vi "SMO.Example.DVRtoRef.vi"(10 "Ref":T1) -> (2 "Ref":u32 format="%08x")   [LabVIEW 2013, in "SMO.Example.lvclass"]
uses:
  SMO.Example.lvclass
  Typedefs/PrivateData--Ref.ctl
  Typedefs/PrivateData--Cluster.ctl
  Typedefs/Configuration--Cluster.ctl
  Typedefs/PublicEvents--Cluster.ctl
  Typedefs/DataChanged--EventData--Cluster.ctl
  Typedefs/ProtectedEvents--Cluster.ctl
  Typedefs/API Inputs--Cluster.ctl
  Typedefs/PumpState--Cluster.ctl
  Typedefs/ValveState--Cluster.ctl
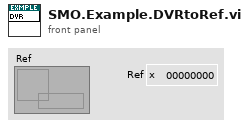
[diagram p1: front panel]
types:
  T1 = typedef "SMO.Example.lvclass/PrivateData--Ref.ctl" = refnum<data-value>
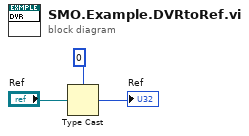
[diagram p0: block diagram]
diagram:
  n1 = Type Cast(type=u32 0 ("Ref"), x="Ref") -> (*(type *) &x=→"Ref":u32)
